vi "LocalisationExample.vi"() -> ()   [LabVIEW 2012]
panel:
  out "Localized String":string
  in  "WordIndex":u32
  in  "LangIndex":u32
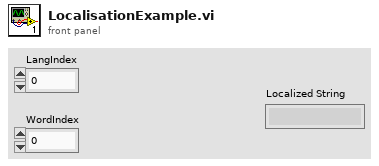
[diagram p1: front panel]
types:
  T1 = cluster{"Indices":u32[], "LocalizedWords":string[][]}
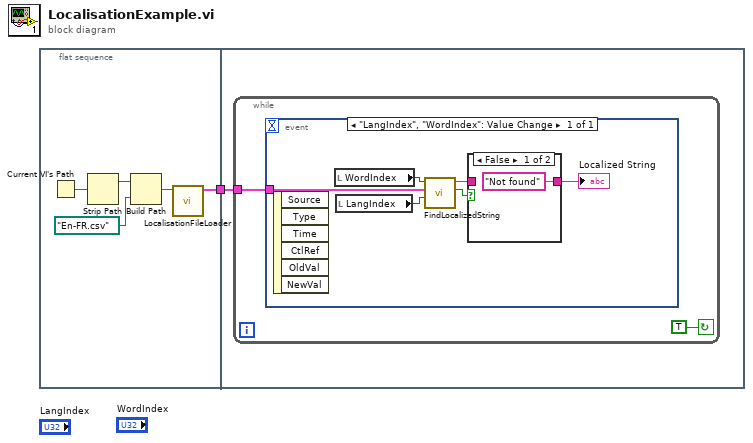
[diagram p0: block diagram]
diagram:
  n1 = flat-sequence {
    tunnel: [w2] -> w1
    tunnel: w1 -> [w7]
    frame #0 {
      n2 = Current VI's Path() -> (path=w6:path)
      n3 = Strip Path(path=w6) -> (stripped path=w5:path)  [unwired: 1 out]
      n4 = Build Path(base path=w5, name or relative path=path "En-FR.csv") -> (appended path=w3:path)
      n5 = call "LocalisationFileLoader.vi"("FilePath"=w3) -> ("LocalisationFileContent[out]"=w2:T1)  [unwired: 10 in]
    }
    frame #1 {
      n6 = while {
        tunnel: w7 -> [w9]
        stop <- TRUE continue-if-true
        n7 = event shown="[0] \"LangIndex\", \"WordIndex\": Value Change" {
          selector: _ -> [_]
          dyn-events: _ -> [_]
          timeout: _ -> [_]
          tunnel: w9 -> [w14]
          event "LangIndex", "WordIndex": Value Change {
            n8 = event-data() -> ()  [unwired: 1 in, 6 out]
            n9 = local read "WordIndex"() -> (w13:u32)
            n10 = local read "LangIndex"() -> (w12:u32)
            n11 = call "FindLocalizedString.vi"("LangIndex"=w12, "LocalizationFileContent"=w14, "WordIndex"=w13) -> ("Found"=w10:bool, "LocalizedString"=w15:string)  [unwired: 7 in]
            n12 = case shown="False" w10 {
              tunnel: w15 -> [_ w17]
              tunnel: ["Not found" w17] -> w11
              frame False {
              }
              frame True {
              }
            }
            "Localized String" <- w11
          }
        }
      }
    }
  }
